vi "JL_Diag_Filter_Faults.vi"(0 "Filter by Count":bool, 5 "Fault Table Entries In":T2[](array[typedef]), 7 "Status":T1) -> (4 "Fault Table Entries Out":T2[](array[typedef]), 6 "Fault Set?":bool)   [LabVIEW 2023]
uses:
  Common/Diagnostics Decode/Type Defs/Diag_FaultTableEntry.ctl
  Common/Diagnostics Decode/Type Defs/Diag_FaultTableStatus.ctl
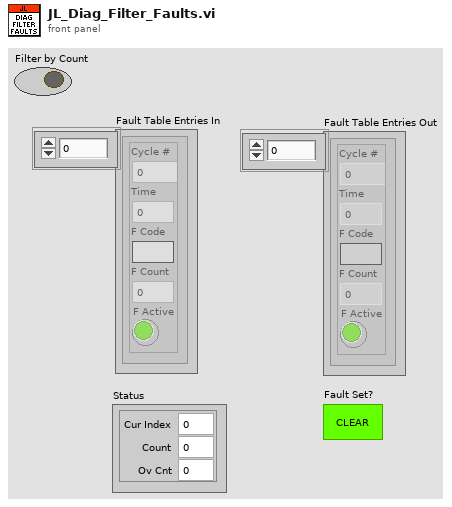
[diagram p1: front panel]
types:
  T1 = typedef "Diag_FaultTableStatus.ctl" = cluster{"Cur Index":u16, "Count":u16, "Ov Cnt":u16}
  T2 = typedef "Diag_FaultTableEntry.ctl" = cluster{"Cycle #":u32, "Time":u32, "F Code":string, "F Count":u16, "F Active":bool}
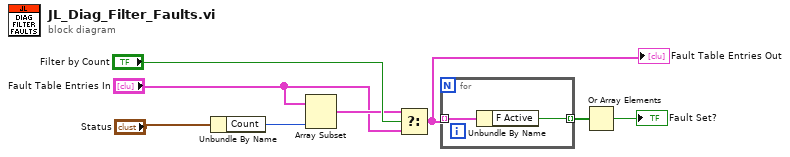
[diagram p0: block diagram]
diagram:
  n1 = Unbundle By Name("Status") -> ("Count"=w6:u16)
  n2 = Array Subset(array="Fault Table Entries In", length=w6) -> (w7:T2[])  [unwired: 1 in]
  n3 = Select(t=w7, s="Filter by Count", f="Fault Table Entries In") -> (s? t:f=w2:T2[])
  "Fault Table Entries Out" <- w2
  n4 = for {
    tunnel: w2 -> [w10] mode=indexing
    tunnel: [w9] -> w5 mode=indexing
    n5 = Unbundle By Name(w10) -> ("F Active"=w9:bool)
  }
  n6 = Or Array Elements(Boolean array=w5) -> (logical OR=→"Fault Set?":bool)
